vi "Main.vi"() -> ()   [LabVIEW 2015]
uses:
  <vilib>/Instr/_visa.llb/VISA Find Search Mode.ctl
  <vilib>/event_ctls.llb/eventvkey.ctl
  <userlib>/_MGI/Application Control/MGI Gray if/MGI Gray if True.vi
  <userlib>/_MGI/Application Control/MGI Disable Enum/MGI Disable Enum (Grayed).vi
  <userlib>/_MGI/Application Control/MGI Disable Enum/MGI Disable Enum (Enabled).vi
panel:
  out "Syringe_defaultSpeed":dbl
  out "message":string
  out "stopFlowIn_StartTime":u32
  out "currentVolume":dbl format="%#_13g"
  out "flowStartTime":u32
  in  "flowingLiquid?":bool=TRUE
  out "Syringe_maxSpeed":dbl
  out "Ref_connectedControls":refnum<vi>[](array[refnum])
  in  "commandString":string
  in  "sendCommand":bool
  in  "SyringeInitialVolumeInitialized?":bool=TRUE
  in  "SyringeAreaInitialized?":bool=TRUE
  out "instrVISA":refnum<visa-resource-name>
  out "Ref_flowControls":refnum<vi>[](array[refnum])
  out "connected?":bool
  in  "connect":bool
  in  "metroMini_ComPort_Strings":string(combo) caption="COM Port"
  in  "syringeSize":dbl(ring) caption="Syringe size / Calibrated area" items=["None"=0.0, "3 mL"=235.60562601155868, "5 mL"=456.92454527165245, "10 mL"=660.519855417254]
  in  "initialVolume":dbl caption="Initial Volume (Max dispensable)" min=0.0 format="%#_g mL"
  in  "enableStopIn":bool caption="Enable"
  in  "stopFlowIn":dbl caption="Stop flow in" format="%.2f min"
  in  "StartFlow":bool
  out "SyringeLevel":dbl(slide) caption="Current Syringe Level" scale=0.0..3.0 scale format="%#_g mL"
  in  "volumeFlowRate":dbl caption="Flow Rate" min=0.0 format="%#_g uL/min"
  # "Connect to Instrument"
  # "Initialize Syringe Parameters"
  # "Control Flow"
  # "Custom Command"
  # "mov # : move distance (mm)\nmov_step # : move number of steps\nstop : stop all movement\ndisable : stop and power down motor"
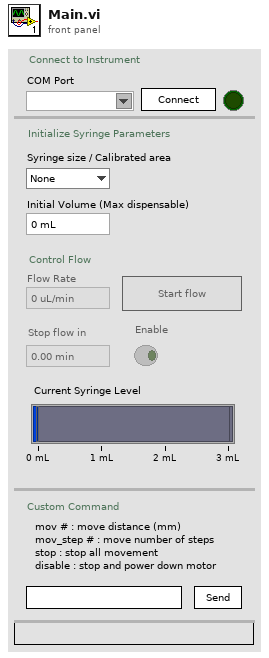
[diagram p1: front panel]
types:
  T1 = enum8{"Enabled", "Disabled", "Disabled and Grayed Out"}
  T2 = typedef "eventvkey.ctl" = enum16{"ASCII", "Enter", "Return", "Shift", "Ctrl", "Alt", "Cmd", "Opt", "Caps", "NumLock", "Clear", "Break", "Up", "Down", "Left", "Right", "Insert", "Delete", "Home", "End", "PageUp", "PageDown", "Escape", "Help", "Pause", "ScrollLock", "F1", "F2", "F3", "F4", "F5", "F6", "F7", "F8", "F9", "F10", "F11", "F12", "F13", "F14", "F15", "F16", "F17", "F18", "F19", "F20", "F21", "F22", "F23", "F24", "Play", "VolumeUp", "VolumeDown", "Mute", "Two Byte Char"}
  T3 = typedef "VISA Find Search Mode.ctl" = u32
  T4 = enum32{"invalid app kind", "Development System", "Run Time System", "Student Edition", "Embedded LabVIEW", "Evaluation", "Custom"}
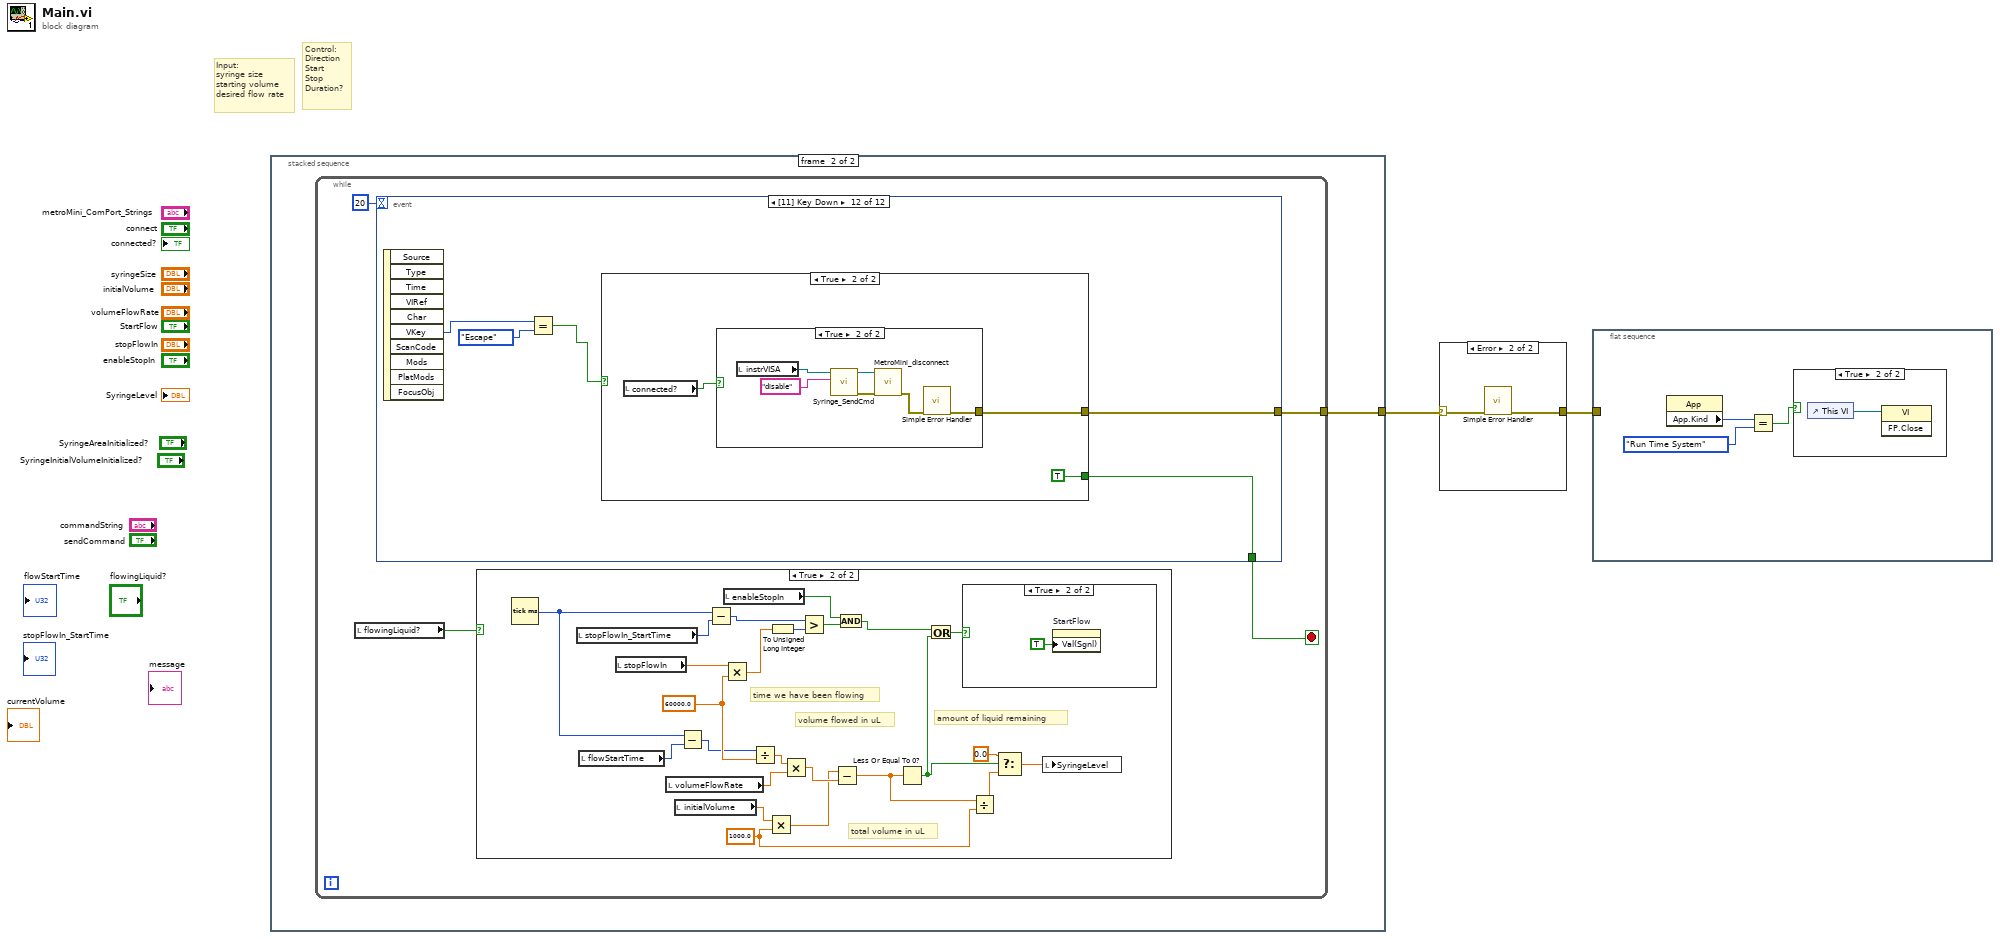
[diagram p0: block diagram]
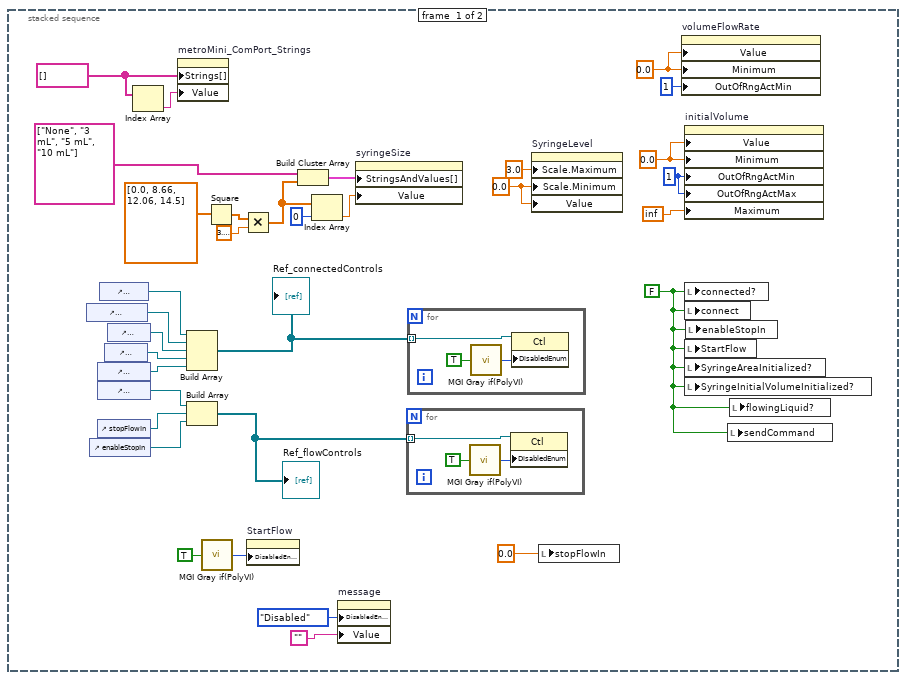
[diagram p4: hidden frame]
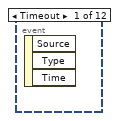
[diagram p7: hidden frame]
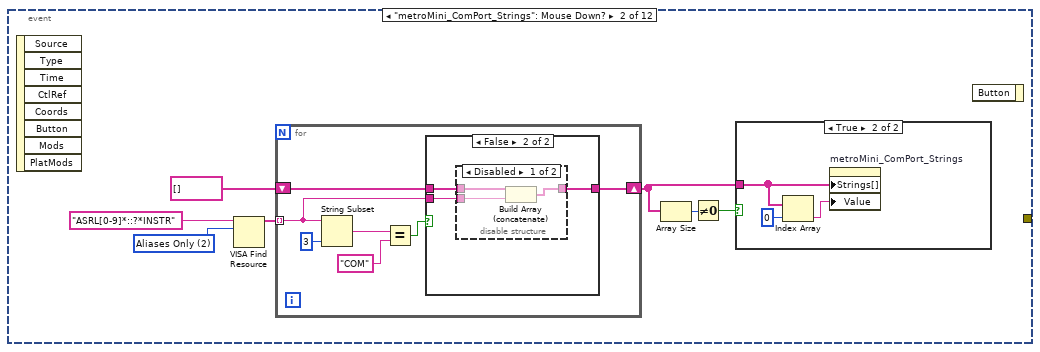
[diagram p8: hidden frame]
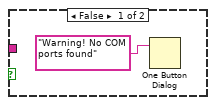
[diagram p9: hidden frame]
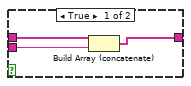
[diagram p10: hidden frame]
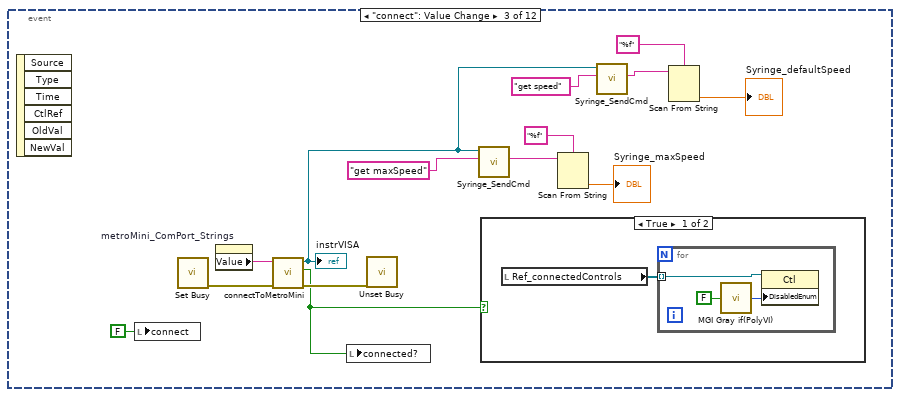
[diagram p12: hidden frame]
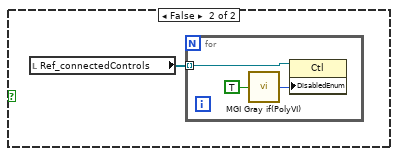
[diagram p13: hidden frame]
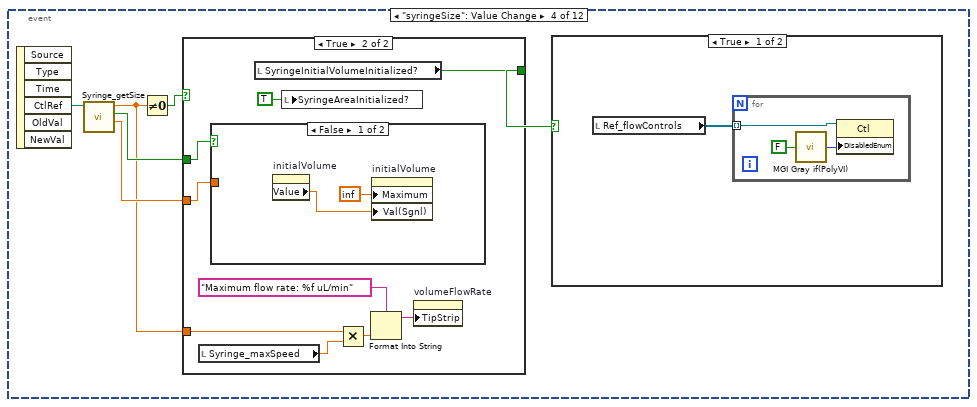
[diagram p14: hidden frame]
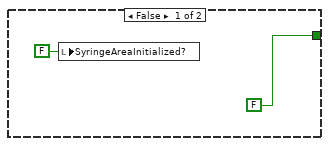
[diagram p15: hidden frame]
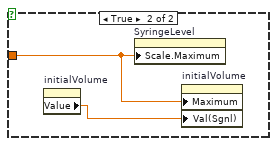
[diagram p16: hidden frame]
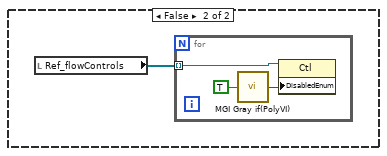
[diagram p17: hidden frame]
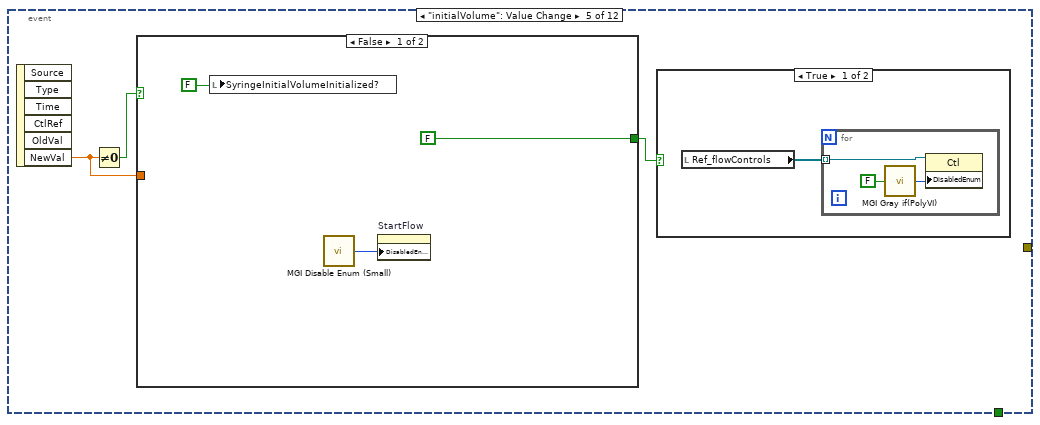
[diagram p18: hidden frame]
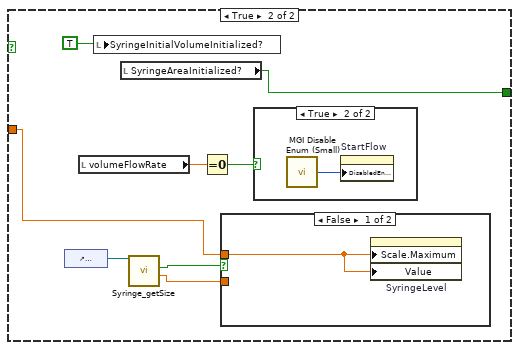
[diagram p19: hidden frame]
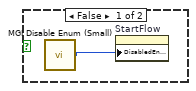
[diagram p20: hidden frame]
diagram:
  # "Control:\nDirection\nStart\nStop\nDuration?"
  # "Input:\nsyringe size\nstarting volume\ndesired flow rate"
  n1 = stacked-sequence {
    tunnel: [_ w42] -> w2
    frame #0 {
      w4 = 0.0 ("Data Entry Limits:Minimum")
      w11 = u8 1 ("Response to Value Outside Limits:Minimum")
      w15 = 0.0 ("Data Entry Limits:Minimum")
      w26 = 0.0 ("Scale.Range:Minimum")
      w9 = FALSE ("True?")
      w28 = string[] [] ("Strings []")
      n2 = control-ref of="sendCommand"() -> (w13:refnum<vi>)
      n3 = control-ref of="enableStopIn"() -> (w34:refnum<vi>)
      n4 = control-ref of="initialVolume"() -> (w32:refnum<vi>)
      n5 = control-ref of="volumeFlowRate"() -> (w33:refnum<vi>)
      n6 = control-ref of="stopFlowIn"() -> (w35:refnum<vi>)
      n7 = control-ref of="commandString"() -> (w14:refnum<vi>)
      n8 = control-ref of="syringeSize"() -> (w31:refnum<vi>)
      n9 = control-ref of="SyringeLevel"() -> (w25:refnum<vi>)
      n10 = Index Array(array=w28) -> (element=w29:string)  [unwired: 1 in]
      n11 = property on="metroMini_ComPort_Strings" class="CmbBox"("Strings[]"=w28, "Value"=w29) -> ()  [unwired: 2 in, 2 out]
      n12 = Build Array(w14, w13, w25, w31, w32) -> (w12:refnum<vi>[])
      "Ref_connectedControls" <- w12
      n13 = Build Array(w33, w35, w34) -> (w30:refnum<vi>[])
      "Ref_flowControls" <- w30
      n14 = call-poly <userlib>:"MGI Gray if(PolyVI).vi"("True?"=TRUE) -> ("Disabled"=w7:T1)
      n15 = Square(x=dbl[] [0.0, 8.66, 12.06, 14.5]) -> (x^2=w22:dbl[])
      n16 = Multiply(x=w22, y=3.141592653589793) -> (x*y=w19:dbl[])
      n17 = property on="StartFlow" class="Bool (strict)"("DisabledEnum"=w7) -> ()  [unwired: 2 in, 2 out]
      n18 = Build Cluster Array(string[] ["None", "3 mL", "5 mL", "10 mL"], w19) -> (w20:cluster{"String":string, dbl}[])
      n19 = Index Array(array=w19, index=0) -> (element=w17:dbl)
      n20 = property on="message" class="Str"("DisabledEnum"=T1."Disabled" ("Disabled"), "Value"="") -> ()  [unwired: 2 in, 2 out]
      n21 = property on="syringeSize" class="Ring (strict)"("StringsAndValues[]"=w20, "Value"=w17) -> ()  [unwired: 2 in, 2 out]
      n22 = for {
        tunnel: w30 -> [w41] mode=indexing
        n23 = call-poly <userlib>:"MGI Gray if(PolyVI).vi"("True?"=TRUE) -> ("Disabled"=w40:T1)
        n24 = property class="Ctl"(reference=w41, "DisabledEnum"=w40) -> ()  [unwired: 1 in, 2 out]
      }
      n25 = for {
        tunnel: w12 -> [w38] mode=indexing
        n26 = call-poly <userlib>:"MGI Gray if(PolyVI).vi"("True?"=TRUE) -> ("Disabled"=w37:T1)
        n27 = property class="Ctl"(reference=w38, "DisabledEnum"=w37) -> ()  [unwired: 1 in, 2 out]
      }
      n28 = property on="SyringeLevel" class="Slide (strict)"("Scale.Maximum"=3.0 ("Scale.Range:Maximum"), "Scale.Minimum"=w26, "Value"=w26) -> ()  [unwired: 2 in, 2 out]
      n29 = local write "stopFlowIn"(0.0 ("volumeFlowRate")) -> ()
      n30 = property on="volumeFlowRate" class="DigNum (strict)"("Value"=w4, "Minimum"=w4, "OutOfRngActMin"=u8 1 ("Response to Value Outside Limits:Minimum")) -> ()  [unwired: 2 in, 2 out]
      n31 = property on="initialVolume" class="DigNum (strict)"("Value"=w15, "Minimum"=w15, "OutOfRngActMin"=w11, "OutOfRngActMax"=w11, "Maximum"=inf) -> ()  [unwired: 2 in, 2 out]
      n32 = local write "connected?"(w9) -> ()
      n33 = local write "connect"(w9) -> ()
      n34 = local write "StartFlow"(w9) -> ()
      n35 = local write "SyringeAreaInitialized?"(w9) -> ()
      n36 = local write "SyringeInitialVolumeInitialized?"(w9) -> ()
      n37 = local write "enableStopIn"(w9) -> ()
      n38 = local write "sendCommand"(w9) -> ()
      n39 = local write "flowingLiquid?"(w9) -> ()
    }
    frame #1 {
      n40 = while {
        tunnel: [w43] -> w42
        stop <- w45 stop-if-true
        n41 = local read "flowingLiquid?"() -> (w44:bool)
        n42 = event shown="[11] Key Down" {
          selector: _ -> [_ _ _ _ _ _ _ _ _ _ _ _]
          dyn-events: _ -> [_ _ _ _ _ _ _ _ _ _ _ _]
          timeout: 20 -> [_ _ _ _ _ _ _ _ _ _ _ _]
          tunnel: [_ _ _ _ _ _ _ _ _ _ TRUE w251] -> w45
          tunnel: [_ _ _ _ _ _ _ _ _ _ _ w249] -> w43
          event Timeout {
            n43 = event-data() -> ()  [unwired: 1 in, 3 out]
          }
          event "metroMini_ComPort_Strings": Mouse Down? {
            w75 = T3 2 items=["Canonical Names Only"=0, "Aliases Only"=2, "Include Matching Aliases"=3, "Include All Aliases"=4] ("Search Mode")
            n44 = event-data() -> ()  [unwired: 1 in, 8 out]
            n45 = VISA Find Resource(10:w75, 11:"ASRL[0-9]*::?*INSTR" ("expression (\"?*\")")) -> (3:w74:string[])  [unwired: 1 in, 2 out]
            n46 = for {
              tunnel: w74 -> [w83] mode=indexing
              shift-right: [w85] -> w78
              shift-left: string[] [] -> [w86]
              n47 = String Subset(string=w83, length (rest)=3 ("length (rest)")) -> (substring=w84:string)  [unwired: 1 in]
              n48 = Equal?(x=w84, y="COM" ("expression (\"?*\")")) -> (x = y?=w87:bool)
              n49 = case shown="False" w87 {
                tunnel: w86 -> [w92 w95]
                tunnel: [w90 w93] -> w85
                tunnel: w83 -> [w91 w94]
                frame True {
                  n50 = Build Array (concatenate)(w92, w91) -> (w90:string[])
                }
                frame False {
                  n51 = disable-structure shown="Disabled" {
                    disable-tunnel: w95 -> [w98 w99]
                    disable-tunnel: w94 -> [w97 _]
                    disable-tunnel: [w96 w99] -> w93
                    frame Disabled {
                      n52 = Build Array (concatenate)(w98, w97) -> (w96:string[])
                    }
                    frame Enabled {
                    }
                  }
                }
              }
            }
            n53 = Array Size(array=w78) -> (size(s)=w72:i32)
            n54 = Not Equal To 0?(x=w72) -> (x != 0?=w77:bool)
            n55 = case shown="True" w77 {
              tunnel: w78 -> [_ w80]
              frame False {
                n56 = One Button Dialog(message="Warning! No COM ports found") -> ()  [unwired: 1 in, 1 out]
              }
              frame True {
                n57 = Index Array(array=w80, index=0) -> (element=w82:string)
                n58 = property on="metroMini_ComPort_Strings" class="CmbBox"("Strings[]"=w80, "Value"=w82) -> ()  [unwired: 2 in, 2 out]
              }
            }
            n59 = event-data() -> ()  [unwired: 2 in, 1 out]
          }
          event "connect": Value Change {
            n60 = event-data() -> ()  [unwired: 1 in, 6 out]
            n61 = local write "connect"(FALSE ("connect")) -> ()
            n62 = call <vilib>:"Set Busy.vi"() -> ("error out"=w113:errorcluster)  [unwired: 10 in, 1 out]
            n63 = property on="metroMini_ComPort_Strings" class="CmbBox"() -> ("Value"=w112:string)  [unwired: 2 in, 2 out]
            n64 = call "connectToMetroMini.vi"("error in"=w113, "visaName"=w112) -> ("error out"=w111:errorcluster, "connected?"=w109:bool, "connectedToInstrument"=w105:refnum<visa-resource-name>)  [unwired: 7 in]
            "instrVISA" <- w105
            n65 = local write "connected?"(w109) -> ()
            n66 = call <vilib>:"Unset Busy.vi"("error in (no error)"=w111) -> ()  [unwired: 10 in, 1 out]
            n67 = call "Syringe_SendCmd.vi"("command"="get maxSpeed", "VISA resource name"=w105) -> ("Message"=w107:string)  [unwired: 7 in, 2 out]
            n68 = case shown="True" w109 {
              frame True {
                n69 = local read "Ref_connectedControls"() -> (w114:refnum<vi>[])
                n70 = for {
                  tunnel: w114 -> [w117] mode=indexing
                  n71 = call-poly <userlib>:"MGI Gray if(PolyVI).vi"("True?"=FALSE) -> ("Disabled"=w116:T1)
                  n72 = property class="Ctl"(reference=w117, "DisabledEnum"=w116) -> ()  [unwired: 1 in, 2 out]
                }
              }
              frame False {
                n73 = local read "Ref_connectedControls"() -> (w118:refnum<vi>[])
                n74 = for {
                  tunnel: w118 -> [w121] mode=indexing
                  n75 = call-poly <userlib>:"MGI Gray if(PolyVI).vi"("True?"=TRUE) -> ("Disabled"=w120:T1)
                  n76 = property class="Ctl"(reference=w121, "DisabledEnum"=w120) -> ()  [unwired: 1 in, 2 out]
                }
              }
            }
            n77 = Scan From String(format string="%f", input string=w107) -> (output 1=→"Syringe_maxSpeed":dbl)  [unwired: 3 in, 3 out]
            n78 = call "Syringe_SendCmd.vi"("command"="get speed", "VISA resource name"=w105) -> ("Message"=w103:string)  [unwired: 7 in, 2 out]
            n79 = Scan From String(format string="%f", input string=w103) -> (output 1=→"Syringe_defaultSpeed":dbl)  [unwired: 3 in, 3 out]
          }
          event "syringeSize": Value Change {
            n80 = event-data() -> ("CtlRef"=w125:refnum<vi>)  [unwired: 1 in, 5 out]
            n81 = call "Syringe_getSize.vi"("Ring Refnum"=w125) -> ("Syringe Size"=w124:dbl, "StandardSize"=w123:bool, "Syringe Area"=w122:dbl)  [unwired: 8 in]
            n82 = Not Equal To 0?(x=w122) -> (x != 0?=w127:bool)
            n83 = case shown="True" w127 {
              tunnel: [FALSE ("SyringeInitialVolumeInitialized?") w137] -> w126
              tunnel: w124 -> [_ w135]
              tunnel: w123 -> [_ w136]
              tunnel: w122 -> [_ w133]
              frame False {
                n84 = local write "SyringeAreaInitialized?"(FALSE ("SyringeAreaInitialized?")) -> ()
              }
              frame True {
                n85 = local read "Syringe_maxSpeed"() -> (w134:dbl)
                n86 = case shown="False" w136 {
                  tunnel: w135 -> [_ w142]
                  frame False {
                    n87 = property on="initialVolume" class="DigNum (strict)"() -> ("Value"=w139:dbl)  [unwired: 2 in, 2 out]
                    n88 = property on="initialVolume" class="DigNum (strict)"("Maximum"=inf, "Val(Sgnl)"=w139) -> ()  [unwired: 2 in, 2 out]
                  }
                  frame True {
                    n89 = property on="initialVolume" class="DigNum (strict)"() -> ("Value"=w141:dbl)  [unwired: 2 in, 2 out]
                    n90 = property on="SyringeLevel" class="Slide (strict)"("Scale.Maximum"=w142) -> ()  [unwired: 2 in, 2 out]
                    n91 = property on="initialVolume" class="DigNum (strict)"("Maximum"=w142, "Val(Sgnl)"=w141) -> ()  [unwired: 2 in, 2 out]
                  }
                }
                n92 = local read "SyringeInitialVolumeInitialized?"() -> (w137:bool)
                n93 = local write "SyringeAreaInitialized?"(TRUE ("SyringeAreaInitialized?")) -> ()
                n94 = Multiply(x=w133, y=w134) -> (x*y=w130:dbl)
                n95 = Format Into String(format string="Maximum flow rate: %f uL/min", w130) -> (resulting string=w132:string)  [unwired: 2 in, 1 out]
                n96 = property on="volumeFlowRate" class="DigNum (strict)"("TipStrip"=w132) -> ()  [unwired: 2 in, 2 out]
              }
            }
            n97 = case shown="True" w126 {
              frame True {
                n98 = local read "Ref_flowControls"() -> (w143:refnum<vi>[])
                n99 = for {
                  tunnel: w143 -> [w146] mode=indexing
                  n100 = call-poly <userlib>:"MGI Gray if(PolyVI).vi"("True?"=FALSE) -> ("Disabled"=w145:T1)
                  n101 = property class="Ctl"(reference=w146, "DisabledEnum"=w145) -> ()  [unwired: 1 in, 2 out]
                }
              }
              frame False {
                n102 = local read "Ref_flowControls"() -> (w147:refnum<vi>[])
                n103 = for {
                  tunnel: w147 -> [w150] mode=indexing
                  n104 = call-poly <userlib>:"MGI Gray if(PolyVI).vi"("True?"=TRUE) -> ("Disabled"=w149:T1)
                  n105 = property class="Ctl"(reference=w150, "DisabledEnum"=w149) -> ()  [unwired: 1 in, 2 out]
                }
              }
            }
          }
          event "initialVolume": Value Change {
            n106 = event-data() -> ("NewVal"=w151:dbl)  [unwired: 1 in, 5 out]
            n107 = Not Equal To 0?(x=w151) -> (x != 0?=w153:bool)
            n108 = case shown="False" w153 {
              tunnel: [FALSE ("SyringeInitialVolumeInitialized?") w163] -> w152
              tunnel: w151 -> [_ w160]
              frame False {
                n109 = local write "SyringeInitialVolumeInitialized?"(FALSE ("SyringeAreaInitialized?")) -> ()
                n110 = call-poly <userlib>:"MGI Disable Enum (Small).vi"() -> ("Disabled & Grayed"=w154:T1)
                n111 = property on="StartFlow" class="Bool (strict)"("DisabledEnum"=w154) -> ()  [unwired: 2 in, 2 out]
              }
              frame True {
                n112 = control-ref of="syringeSize"() -> (w162:refnum<vi>)
                n113 = local read "volumeFlowRate"() -> (w157:dbl)
                n114 = local write "SyringeInitialVolumeInitialized?"(TRUE ("SyringeAreaInitialized?")) -> ()
                n115 = local read "SyringeAreaInitialized?"() -> (w163:bool)
                n116 = call "Syringe_getSize.vi"("Ring Refnum"=w162) -> ("Syringe Size"=w159:dbl, "StandardSize"=w161:bool)  [unwired: 8 in, 1 out]
                n117 = Equal To 0?(x=w157) -> (x = 0?=w158:bool)
                n118 = case shown="False" w161 {
                  tunnel: w160 -> [w167 w170]
                  tunnel: w159 -> [_ w169]
                  frame False {
                    n119 = property on="SyringeLevel" class="Slide (strict)"("Scale.Maximum"=w167, "Value"=w167) -> ()  [unwired: 2 in, 2 out]
                  }
                  frame True {
                    n120 = Less Or Equal?(x=w170, y=w169) -> (x <= y?=w171:bool)
                    n121 = Select(t=w170, s=w171, f=w169) -> (s? t:f=w168:dbl)
                    n122 = local write "initialVolume"(w168) -> ()
                    n123 = local write "SyringeLevel"(w168) -> ()
                  }
                }
                n124 = case shown="True" w158 {
                  frame False {
                    n125 = call-poly <userlib>:"MGI Disable Enum (Small).vi"() -> ("Enabled"=w165:T1)
                    n126 = property on="StartFlow" class="Bool (strict)"("DisabledEnum"=w165) -> ()  [unwired: 2 in, 2 out]
                  }
                  frame True {
                    n127 = call-poly <userlib>:"MGI Disable Enum (Small).vi"() -> ("Disabled & Grayed"=w166:T1)
                    n128 = property on="StartFlow" class="Bool (strict)"("DisabledEnum"=w166) -> ()  [unwired: 2 in, 2 out]
                  }
                }
              }
            }
            n129 = case shown="True" w152 {
              frame True {
                n130 = local read "Ref_flowControls"() -> (w172:refnum<vi>[])
                n131 = for {
                  tunnel: w172 -> [w175] mode=indexing
                  n132 = call-poly <userlib>:"MGI Gray if(PolyVI).vi"("True?"=FALSE) -> ("Disabled"=w174:T1)
                  n133 = property class="Ctl"(reference=w175, "DisabledEnum"=w174) -> ()  [unwired: 1 in, 2 out]
                }
              }
              frame False {
                n134 = local read "Ref_flowControls"() -> (w176:refnum<vi>[])
                n135 = for {
                  tunnel: w176 -> [w179] mode=indexing
                  n136 = call-poly <userlib>:"MGI Gray if(PolyVI).vi"("True?"=TRUE) -> ("Disabled"=w178:T1)
                  n137 = property class="Ctl"(reference=w179, "DisabledEnum"=w178) -> ()  [unwired: 1 in, 2 out]
                }
              }
            }
          }
          event "volumeFlowRate": Value Change {
            n138 = event-data() -> ("NewVal"=w184:dbl)  [unwired: 1 in, 5 out]
            n139 = local read "Syringe_maxSpeed"() -> (w186:dbl)
            n140 = local read "syringeSize"() -> (w185:dbl)
            n141 = Multiply(x=w186, y=w185) -> (x*y=w183:dbl)
            n142 = In Range and Coerce(upper limit=w183, x=w184, lower limit=0.0) -> (coerced(x)=w181:dbl)  [unwired: 1 out]
            n143 = local write "volumeFlowRate"(w181) -> ()
            n144 = Equal To 0?(x=w181) -> (x = 0?=w180:bool)
            n145 = case shown="False" w180 {
              frame False {
                n146 = call-poly <userlib>:"MGI Disable Enum (Small).vi"() -> ("Enabled"=w187:T1)
                n147 = property on="StartFlow" class="Bool (strict)"("DisabledEnum"=w187) -> ()  [unwired: 2 in, 2 out]
              }
              frame True {
                n148 = call-poly <userlib>:"MGI Disable Enum (Small).vi"() -> ("Disabled & Grayed"=w188:T1)
                n149 = property on="StartFlow" class="Bool (strict)"("DisabledEnum"=w188) -> ()  [unwired: 2 in, 2 out]
              }
            }
          }
          event "enableStopIn": Value Change {
            n150 = event-data() -> ("NewVal"=w191:bool)  [unwired: 1 in, 5 out]
            n151 = local read "flowingLiquid?"() -> (w190:bool)
            n152 = And(x=w191, y=w190) -> (x .and. y?=w189:bool)
            n153 = case shown="True" w189 {
              frame False {
              }
              frame True {
                n154 = Tick Count (ms)() -> (millisecond timer value=w192:u32)
                n155 = local write "stopFlowIn_StartTime"(w192) -> ()
              }
            }
          }
          event "stopFlowIn": Value Change {
            n156 = event-data() -> ("OldVal"=w197:dbl, "NewVal"=w196:dbl)  [unwired: 1 in, 4 out]
            n157 = local read "flowingLiquid?"() -> (w194:bool)
            n158 = Not Equal?(x=w197, y=w196) -> (x != y?=w195:bool)
            n159 = And(x=w195, y=w194) -> (x .and. y?=w193:bool)
            n160 = case shown="True" w193 {
              frame False {
              }
              frame True {
                n161 = Tick Count (ms)() -> (millisecond timer value=w198:u32)
                n162 = local write "stopFlowIn_StartTime"(w198) -> ()
              }
            }
          }
          event "StartFlow": Value Change {
            n163 = event-data() -> ()  [unwired: 1 in, 6 out]
            n164 = local read "flowingLiquid?"() -> (w200:bool)
            n165 = case shown="True" w200 {
              frame True {
                # "Stop the flow."
                n166 = local read "SyringeLevel"() -> (w201:dbl)
                n167 = local read "instrVISA"() -> (w209:refnum<visa-resource-name>)
                n168 = local write "flowingLiquid?"(FALSE ("flowingLiquid?")) -> ()
                n169 = property on="StartFlow" class="Bool (strict)"("BoolText.Text"="Start flow" ("Boolean Text.Text")) -> ()  [unwired: 2 in, 2 out]
                n170 = local write "message"("" ("message")) -> ()
                n171 = call "Syringe_SendCmd.vi"("command"="disable", "VISA resource name"=w209) -> ()  [unwired: 7 in, 3 out]
                n172 = local read "Syringe_defaultSpeed"() -> (w202:dbl)
                n173 = property on="initialVolume" class="DigNum (strict)"("Val(Sgnl)"=w201) -> ()  [unwired: 2 in, 2 out]
                n174 = call-poly <userlib>:"MGI Disable Enum (Small).vi"() -> ("Enabled"=w206:T1)
                n175 = local read "instrVISA"() -> (w203:refnum<visa-resource-name>)
                n176 = property on="volumeFlowRate" class="DigNum (strict)"("DisabledEnum"=w206) -> ()  [unwired: 2 in, 2 out]
                n177 = Format Into String(format string="speed %f", w202) -> (resulting string=w205:string)  [unwired: 2 in, 1 out]
                n178 = call "Syringe_SendCmd.vi"("command"=w205, "VISA resource name"=w203) -> ()  [unwired: 7 in, 3 out]
              }
              frame False {
                # "Start liquid flow"
                n179 = call-poly <userlib>:"MGI Disable Enum (Small).vi"() -> ("Disabled & Grayed"=w219:T1)
                n180 = local read "volumeFlowRate"() -> (w215:dbl)
                n181 = local read "syringeSize"() -> (w218:dbl)
                n182 = property on="volumeFlowRate" class="DigNum (strict)"("DisabledEnum"=w219) -> ()  [unwired: 2 in, 2 out]
                n183 = Divide(x=w215, y=w218) -> (x/y=w217:dbl)
                n184 = Format Into String(format string="speed %f", w217) -> (resulting string=w214:string)  [unwired: 2 in, 1 out]
                n185 = local read "instrVISA"() -> (w213:refnum<visa-resource-name>)
                n186 = Tick Count (ms)() -> (millisecond timer value=w221:u32)
                n187 = call "Syringe_SendCmd.vi"("command"=w214, "VISA resource name"=w213) -> ("VISA resource out"=w212:refnum<visa-resource-name>)  [unwired: 7 in, 2 out]
                n188 = local write "flowStartTime"(w221) -> ()
                n189 = local write "stopFlowIn_StartTime"(w221) -> ()
                n190 = local write "message"("Liquid flowing" ("message")) -> ()
                n191 = local write "flowingLiquid?"(TRUE ("flowingLiquid?")) -> ()
                n192 = property on="StartFlow" class="Bool (strict)"("BoolText.Text"="Stop flow" ("Boolean Text.Text")) -> ()  [unwired: 2 in, 2 out]
                n193 = call "Syringe_SendCmd.vi"("command"="fwd", "VISA resource name"=w212) -> ()  [unwired: 7 in, 3 out]
              }
            }
            n194 = local write "StartFlow"(FALSE ("StartFlow")) -> ()
          }
          event "sendCommand": Value Change {
            n195 = event-data() -> ()  [unwired: 1 in, 6 out]
            n196 = local read "commandString"() -> (w225:string)
            n197 = local read "flowingLiquid?"() -> (w228:bool)
            n198 = case shown="True" w228 {
              tunnel: [w230 w236] -> w227
              tunnel: ["" ""] -> w226
              tunnel: w225 -> [w231 w234]
              frame False {
                n199 = local read "instrVISA"() -> (w232:refnum<visa-resource-name>)
                n200 = call "Syringe_SendCmd.vi"("command"=w231, "VISA resource name"=w232) -> ("Message"=w230:string)  [unwired: 7 in, 2 out]
              }
              frame True {
                n201 = case shown="\"disable\", \"stop\"" w234 {
                  selector: w234 -> [w238 _ _]
                  tunnel: [w237 "Command not allowed while flowing." ("Message") "Stopping..." ("Message")] -> w236
                  frame "speed" {
                    n202 = local read "instrVISA"() -> (w239:refnum<visa-resource-name>)
                    n203 = call "Syringe_SendCmd.vi"("command"=w238, "VISA resource name"=w239) -> ("Message"=w237:string)  [unwired: 7 in, 2 out]
                  }
                  frame Default {
                  }
                  frame "disable", "stop" {
                    n204 = property on="StartFlow" class="Bool (strict)"("Val(Sgnl)"=TRUE ("Value (Signaling)")) -> ()  [unwired: 2 in, 2 out]
                  }
                }
              }
            }
            n205 = local write "sendCommand"(FALSE ("sendCommand")) -> ()
            n206 = local write "commandString"(w226) -> ()
            n207 = local write "message"(w227) -> ()
          }
          event Panel Close {
            n208 = event-data() -> ()  [unwired: 1 in, 4 out]
            n209 = local read "connected?"() -> (w244:bool)
            n210 = case shown="True" w244 {
              frame False {
              }
              frame True {
                n211 = local read "instrVISA"() -> (w248:refnum<visa-resource-name>)
                n212 = call "Syringe_SendCmd.vi"("command"="disable", "VISA resource name"=w248) -> ("error out"=w246:errorcluster, "VISA resource out"=w245:refnum<visa-resource-name>)  [unwired: 7 in, 1 out]
                n213 = call "MetroMini_disconnect.vi"("error in (no error)"=w246, "VISA resource name"=w245) -> ()  [unwired: 9 in, 1 out]
              }
            }
          }
          event Key Down {
            n214 = event-data() -> ("VKey"=w253:T2)  [unwired: 1 in, 9 out]
            n215 = Equal?(x=w253, y=eventvkey."Escape" ("VKey")) -> (x = y?=w250:bool)
            n216 = case shown="True" w250 {
              tunnel: [FALSE TRUE] -> w251
              tunnel: [_ w255] -> w249
              frame False {
              }
              frame True {
                n217 = local read "connected?"() -> (w256:bool)
                n218 = case shown="True" w256 {
                  tunnel: [_ w258] -> w255
                  frame False {
                  }
                  frame True {
                    n219 = local read "instrVISA"() -> (w263:refnum<visa-resource-name>)
                    n220 = call "Syringe_SendCmd.vi"("command"="disable", "VISA resource name"=w263) -> ("error out"=w261:errorcluster, "VISA resource out"=w260:refnum<visa-resource-name>)  [unwired: 7 in, 1 out]
                    n221 = call "MetroMini_disconnect.vi"("error in (no error)"=w261, "VISA resource name"=w260) -> ("error out"=w259:errorcluster)  [unwired: 9 in]
                    n222 = call <vilib>:"Simple Error Handler.vi"("error in (no error)"=w259) -> ("error out"=w258:errorcluster)  [unwired: 4 in, 4 out]
                  }
                }
              }
            }
          }
        }
        n223 = case shown="True" w44 {
          frame False {
          }
          frame True {
            w51 = 1000.0 ("y")
            w65 = 60000.0
            # "amount of liquid remaining"
            # "time we have been flowing"
            # "total volume in uL"
            # "volume flowed in uL"
            n224 = Tick Count (ms)() -> (millisecond timer value=w55:u32)
            n225 = local read "stopFlowIn_StartTime"() -> (w70:u32)
            n226 = local read "flowStartTime"() -> (w56:u32)
            n227 = local read "stopFlowIn"() -> (w69:dbl)
            n228 = local read "volumeFlowRate"() -> (w63:dbl)
            n229 = local read "initialVolume"() -> (w62:dbl)
            n230 = Subtract(x=w55, y=w56) -> (x-y=w54:u32)
            n231 = Subtract(x=w55, y=w70) -> (x-y=w66:u32)
            n232 = local read "enableStopIn"() -> (w57:bool)
            n233 = Multiply(x=w69, y=w65) -> (x*y=w67:dbl)
            n234 = Divide(x=w54, y=w65) -> (x/y=w64:dbl)
            n235 = Multiply(x=w62, y=w51) -> (x*y=w60:dbl)
            n236 = To Unsigned Long Integer(number=w67) -> (unsigned 32bit integer=w68:u32)
            n237 = Multiply(x=w64, y=w63) -> (x*y=w61:dbl)
            n238 = Greater?(x=w66, y=w68) -> (0:w58:bool)
            n239 = Subtract(x=w60, y=w61) -> (x-y=w52:dbl)
            n240 = And(x=w57, y=w58) -> (x .and. y?=w53:bool)
            n241 = Less Or Equal To 0?(x=w52) -> (x <= 0?=w49:bool)
            n242 = Or(x=w53, y=w49) -> (x .or. y?=w59:bool)
            n243 = case shown="True" w59 {
              frame False {
              }
              frame True {
                n244 = property on="StartFlow" class="Bool (strict)"("Val(Sgnl)"=TRUE ("Value (Signaling)")) -> ()  [unwired: 2 in, 2 out]
              }
            }
            n245 = Divide(x=w52, y=w51) -> (x/y=w50:dbl)
            n246 = Select(t=0.0, s=w49, f=w50) -> (s? t:f=w47:dbl)
            n247 = local write "SyringeLevel"(w47) -> ()
          }
        }
      }
    }
  }
  n248 = case shown="Error" w2 {
    selector: w2 -> [w264 w266]
    tunnel: [w264 w265] -> w1
    frame No Error {
    }
    frame Error {
      n249 = call <vilib>:"Simple Error Handler.vi"("error in (no error)"=w266) -> ("error out"=w265:errorcluster)  [unwired: 4 in, 4 out]
    }
  }
  n250 = flat-sequence {
    tunnel: w1 -> [_]
    frame #0 {
      n251 = property class="App"() -> ("App.Kind"=w269:T4)  [unwired: 2 in, 2 out]
      n252 = Equal?(x=w269, y=T4."Run Time System" ("Application:Kind")) -> (x = y?=w267:bool)
      n253 = case shown="True" w267 {
        frame False {
        }
        frame True {
          n254 = control-ref of="This VI"() -> (w270:refnum<vi>)
          n255 = invoke class="VI" method="FP.Close"(reference=w270) -> ()  [unwired: 2 in, 3 out]
        }
      }
    }
  }
